vi "TestCloneAPI.vi"() -> ()   [LabVIEW 2014, in "DigitizerModule.lvlib"]
uses:
  DigitizerModule.lvlib
  DigitizerPlugins/DigitizerBaseClass/Typedefs/WfrmAttributes.ctl
  TestInfo.ctl
  <userlib>/NIST/ModuleAdminLib/CloneRegistration/CloneRegistration.lvclass
  <userlib>/NIST/ModuleAdminLib/ModuleAdmin/ModuleAdmin.lvclass/ModuleAdmin.ctl
  <userlib>/NIST/ModuleAdminLib/ModuleAdmin/ModuleAdmin.lvclass
  PublicAPI/Arguments/Broadcasts/clDidInit.ctl
  PublicAPI/Arguments/Requests/clStopArgument.ctl
  <userlib>/NIST/ModuleAdminLib/ModuleAdmin/Accessors/Read CloneRegRef.vi
  <userlib>/NIST/ModuleAdminLib/ModuleAdmin/Accessors/Write CloneRegRef.vi
  DigitizerPlugins/DigitizerBaseClass/DigitizerBase.lvclass
panel:
  out "Attributes":T1[][](array[typedef])
  out "Timing":cluster{"Time Stamp":timestamp, "dt":dbl}[][](array[cluster])
  in  "btnAbort":bool
  in  "btnClear":bool
  in  "btnCfgTrig":bool
  in  "btnCfgAquis":bool
  in  "btnCfgChan":bool
  out "Waveform Chart":waveform(dbl)[](graph)
  in  "btnInitialize":bool
  in  "btnReadWfrm":bool
  in  "btnFetch":bool
  in  "btnPref":bool
  in  "Show Panel":bool=TRUE
  in  "Plugin Type":u16(ring) items=["IVI Digitizer", "Analyse Waveforms", "Debug", "Ni DaqMx Digitizer", "PMU Cal", "(obsolete)", "Simulation"]
  in  "btnLoadPlugin":bool
  out "Path":path
  in  "btnRequestINIPath":bool
  in  "btnRemove":bool
  out "Status Log":string
  out "Active Modules (Array)":string[](array[string])
  in  "btnAdd":bool
  in  "btnStop":bool
  in  "Select Module":i32(ring)=-1 caption="Select Module to send Request" items=["All"=-1, "4140002"=4140002]
  # "Hidden"
  # "Visible"
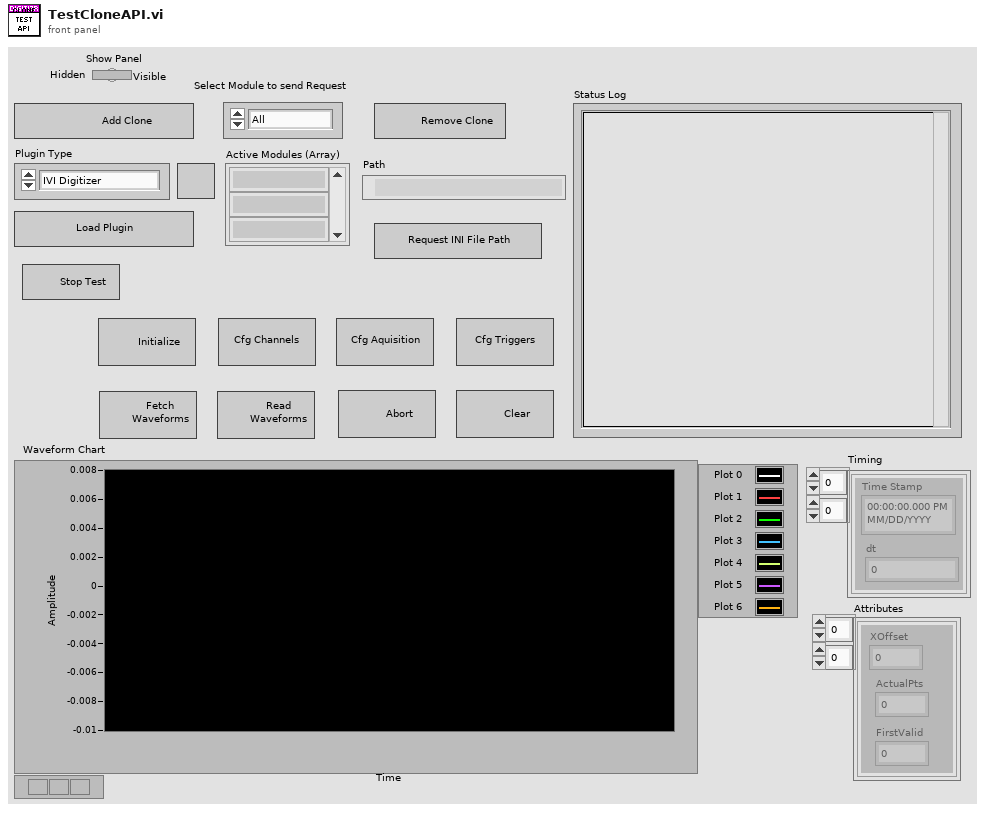
[diagram p1: front panel]
types:
  T1 = typedef "DigitizerPlugins.lvlib/DigitizerBase.lvclass/WfrmAttributes.ctl" = cluster{"XOffset":dbl, "ActualPts":i64, "FirstValid":i64}
  T2 = typedef "DigitizerModule.lvlib/TestInfo.ctl" = cluster{"PluginIniFilePaths":path[]}
  T3 = typedef "DigitizerModule.lvlib/clBroadcastEvents.ctl" = cluster{"DidInit":refnum<user-event>, "StatusUpdate":refnum<user-event>, "ErrorReport":refnum<user-event>, "DidStop":refnum<user-event>, "PathToINI":refnum<user-event>, "Channels":refnum<user-event>, "Acq":refnum<user-event>, "Trigger":refnum<user-event>, "Waveforms":refnum<user-event>}
  T4 = typedef "DigitizerModule.lvlib/clDidInit.ctl" = cluster{"Init?":bool, "ModuleAdmin":refnum<class "ModuleAdmin.lvclass">}
  T5 = typedef "DigitizerModule.lvlib/clStopArgument.ctl" = cluster{"Exit via Stop Module Req?":bool, "Wait for Module to stop?":bool, "ModuleAdmin":refnum<class "ModuleAdmin.lvclass">}
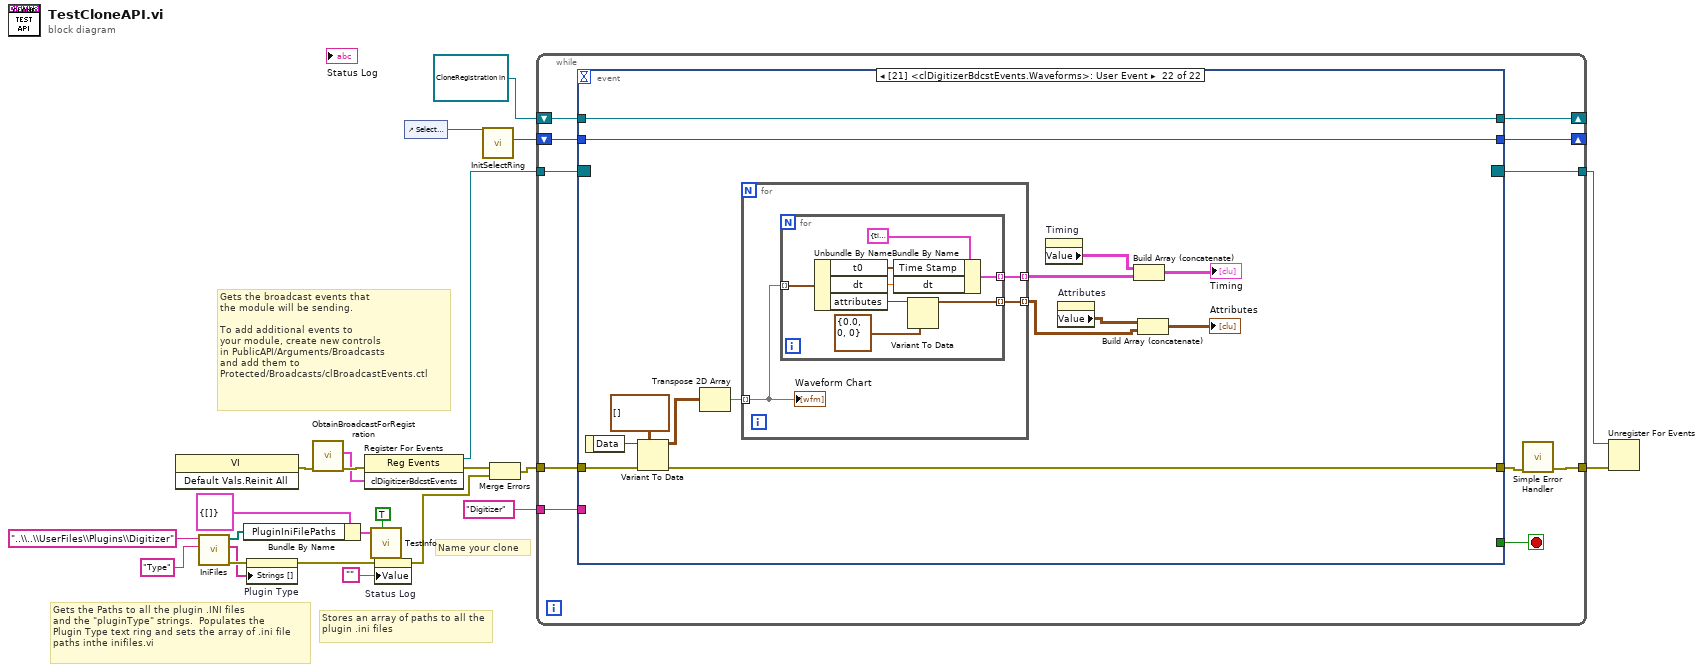
[diagram p0: block diagram]
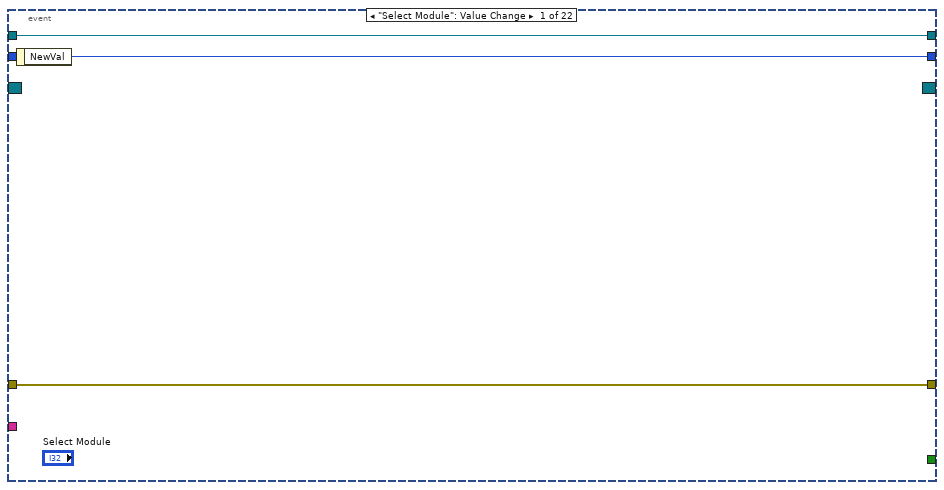
[diagram p2: hidden frame]
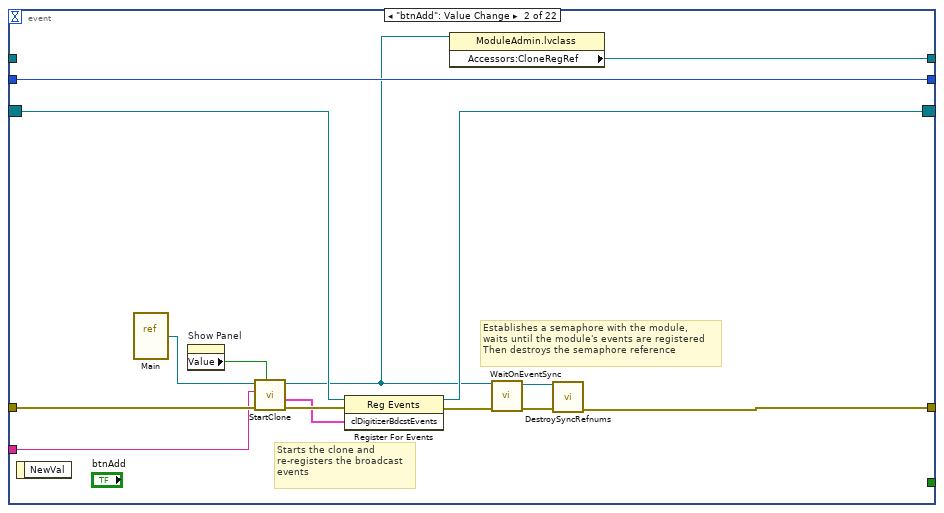
[diagram p3: hidden frame]
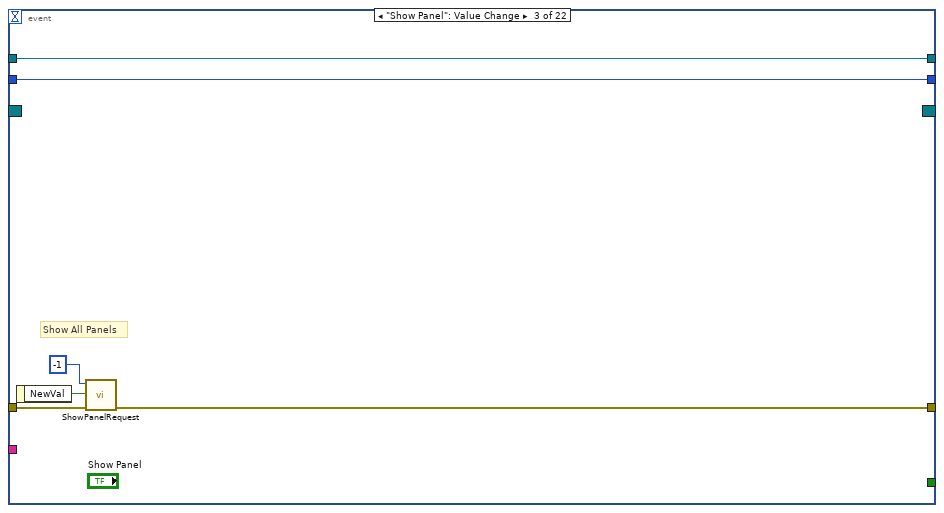
[diagram p4: hidden frame]
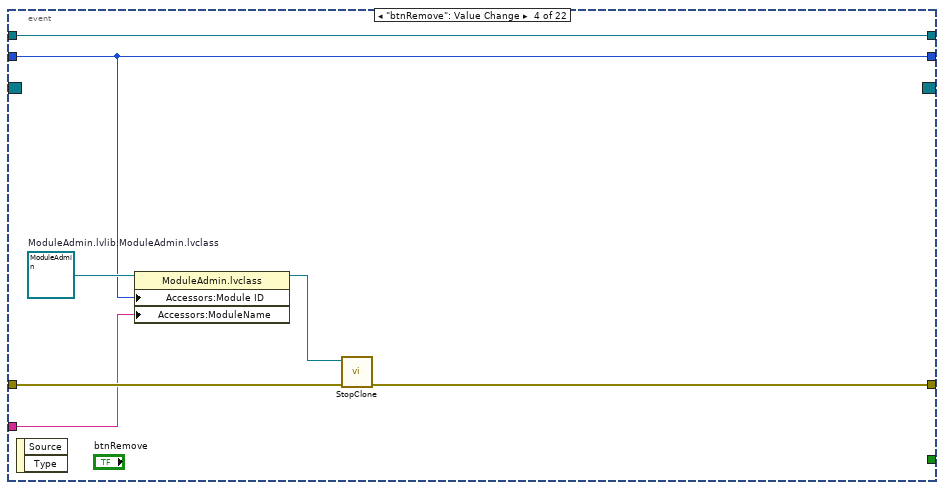
[diagram p5: hidden frame]
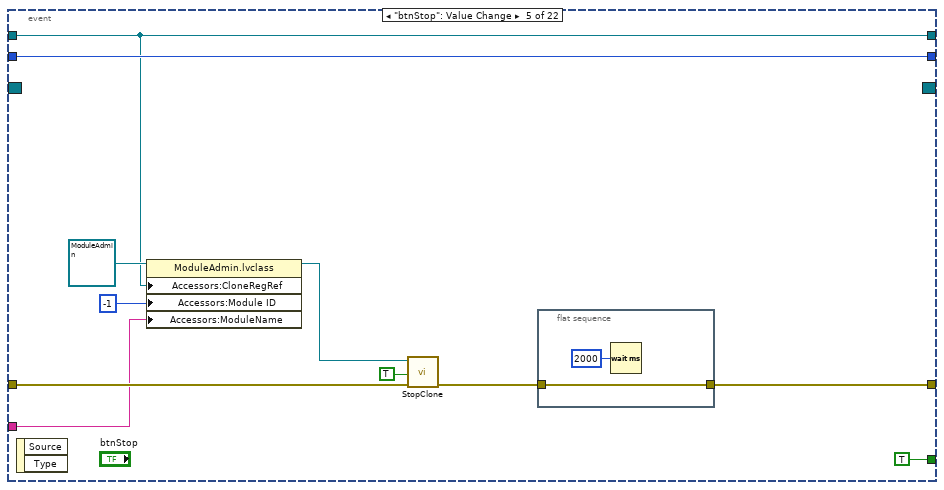
[diagram p6: hidden frame]
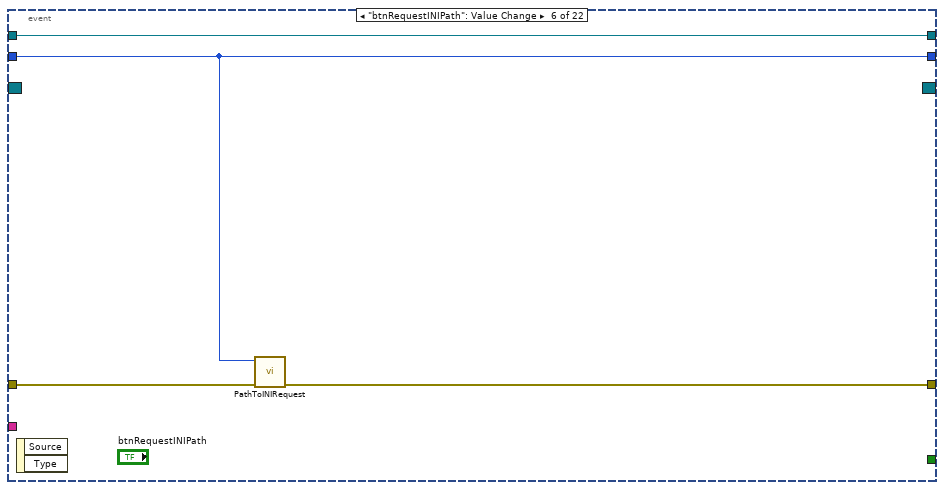
[diagram p7: hidden frame]
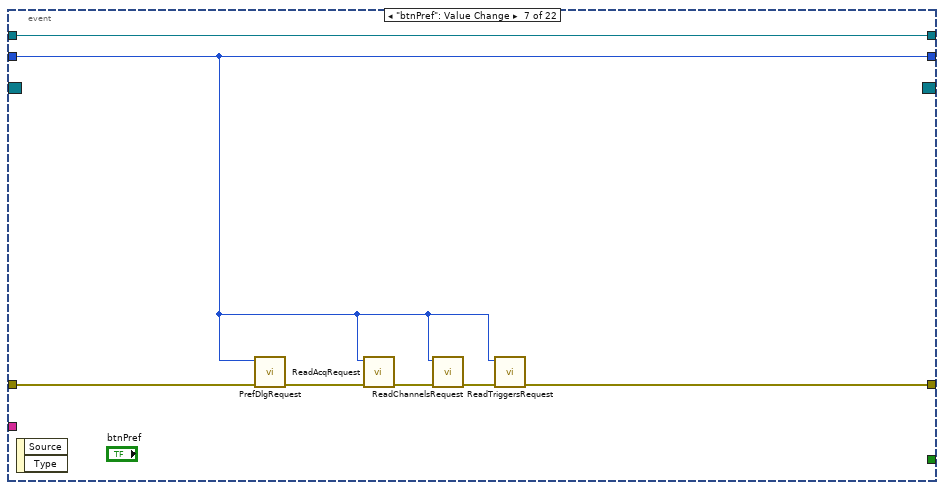
[diagram p8: hidden frame]
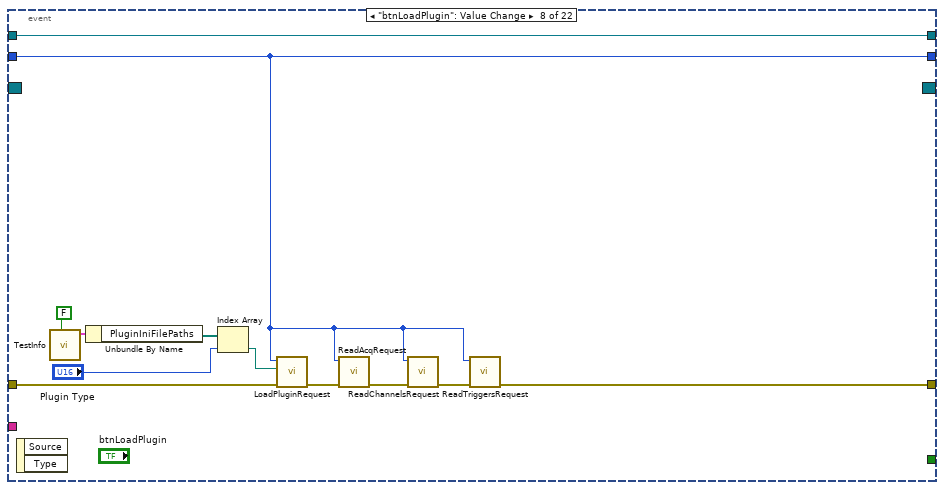
[diagram p9: hidden frame]
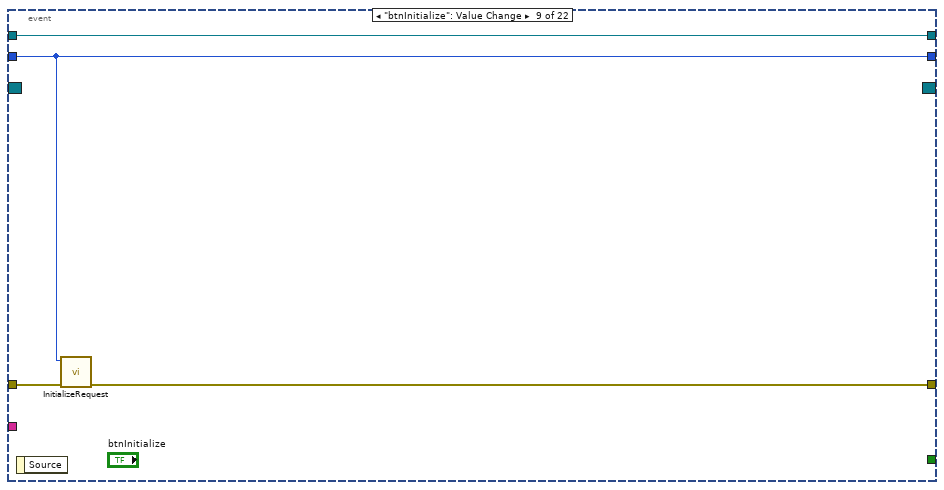
[diagram p10: hidden frame]
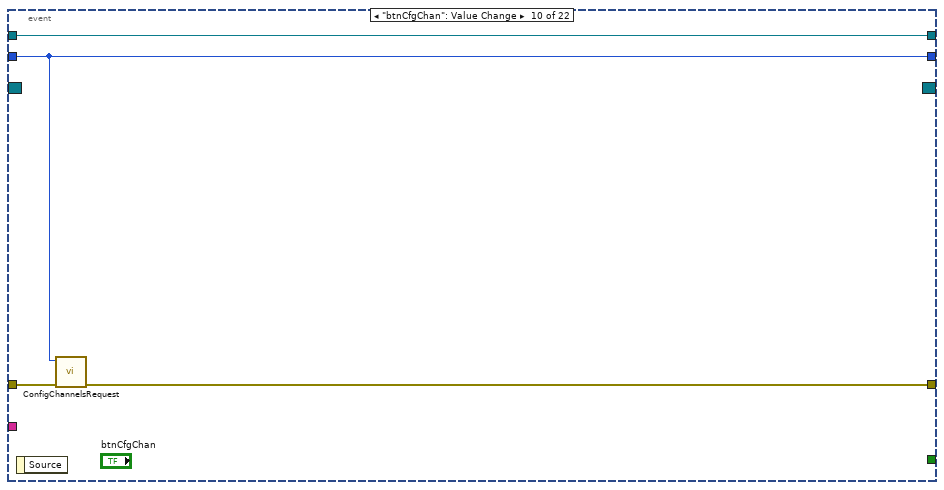
[diagram p11: hidden frame]
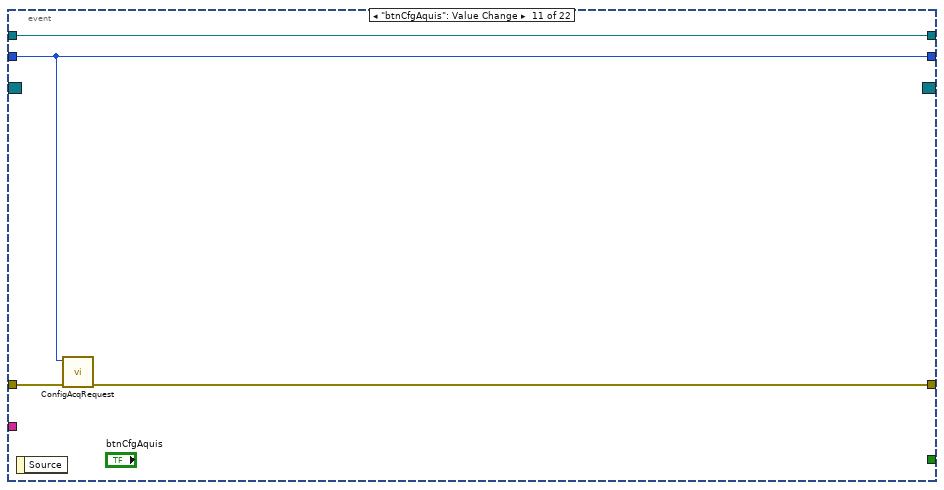
[diagram p12: hidden frame]
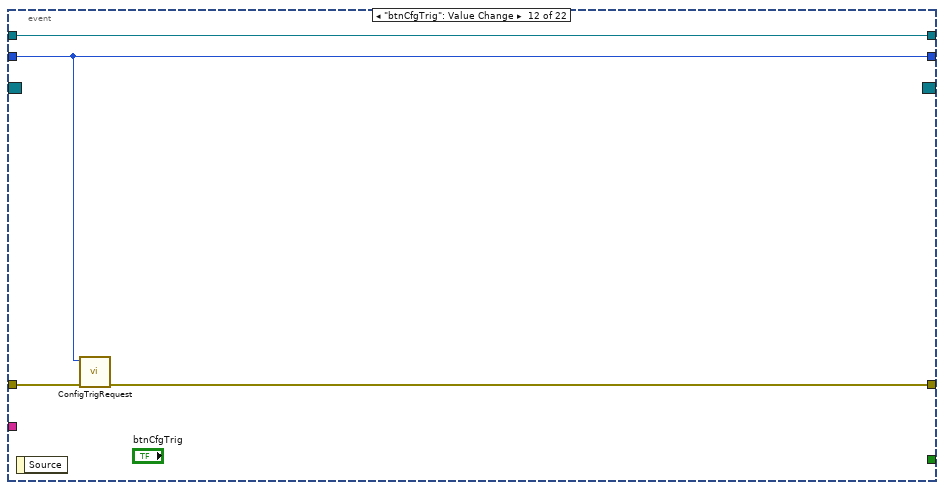
[diagram p13: hidden frame]
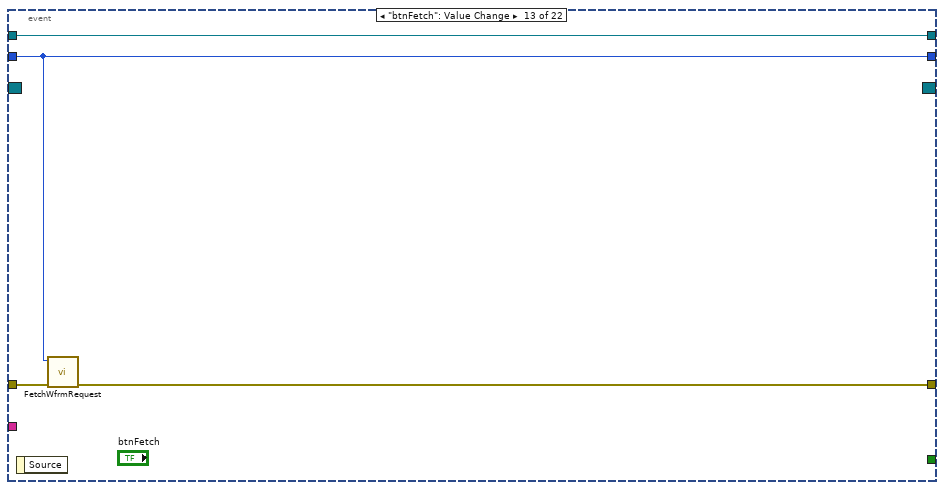
[diagram p14: hidden frame]
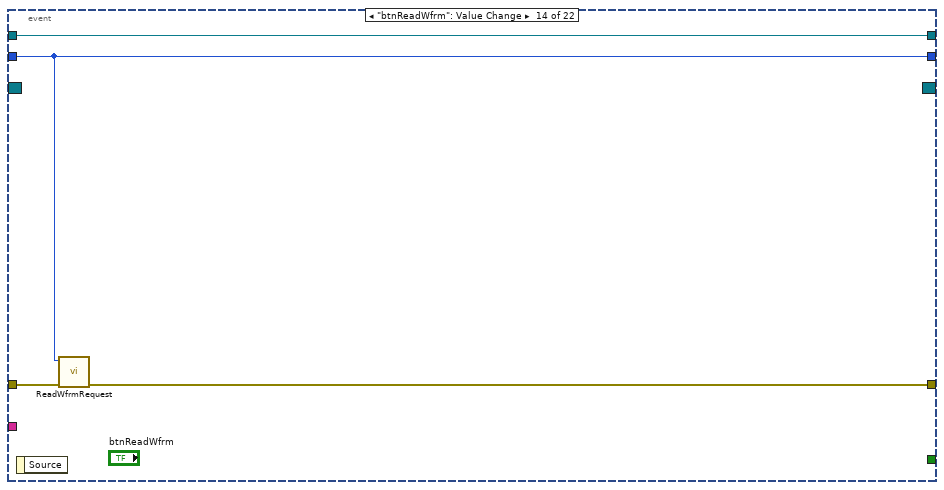
[diagram p15: hidden frame]
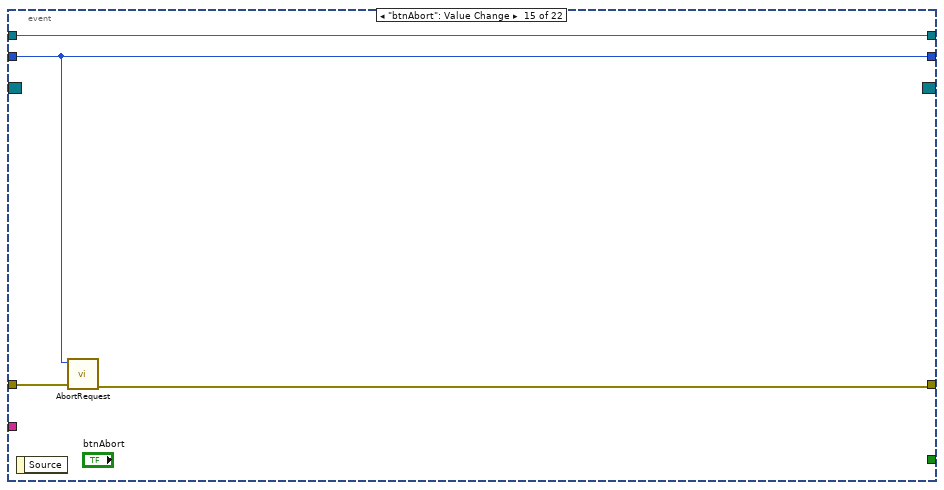
[diagram p16: hidden frame]
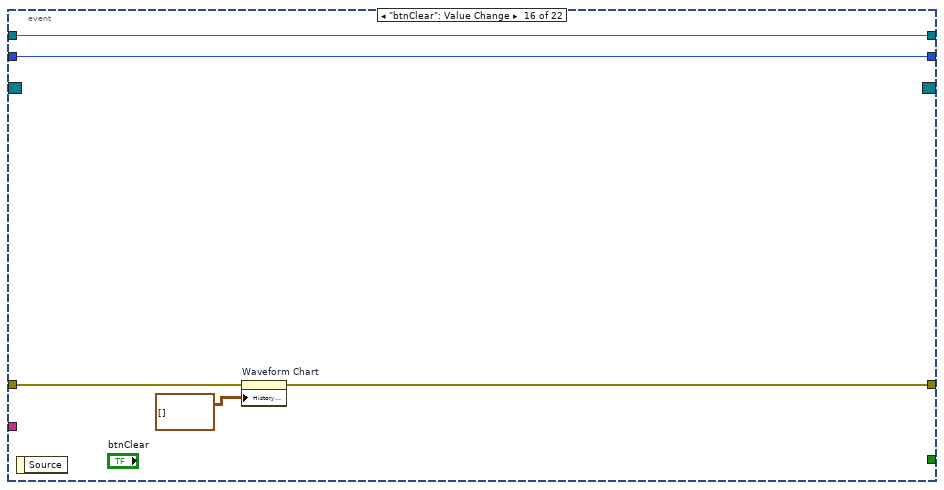
[diagram p17: hidden frame]
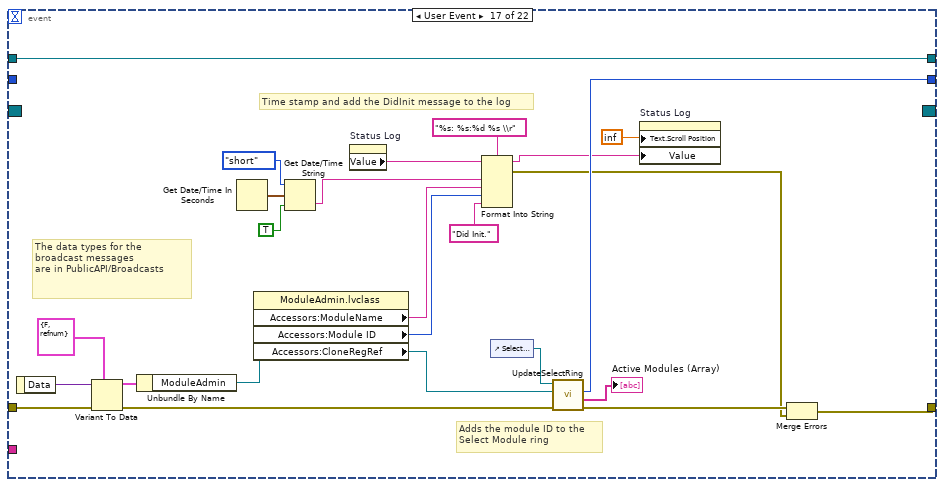
[diagram p18: hidden frame]
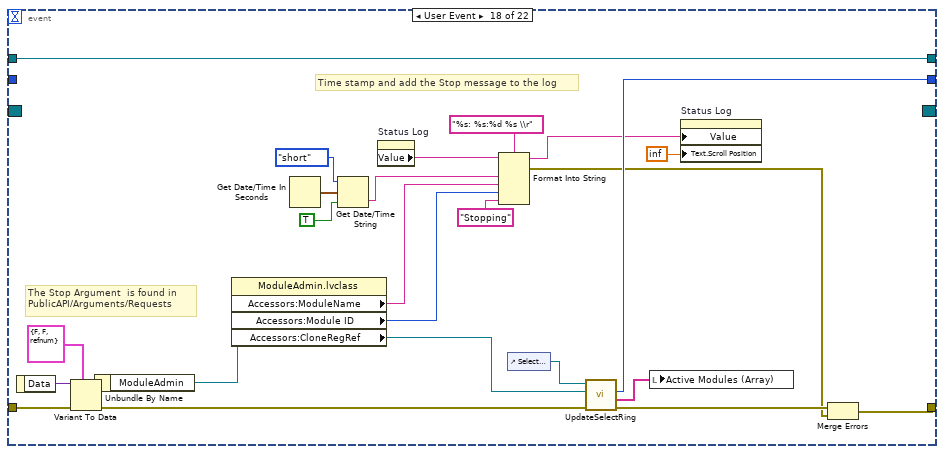
[diagram p19: hidden frame]
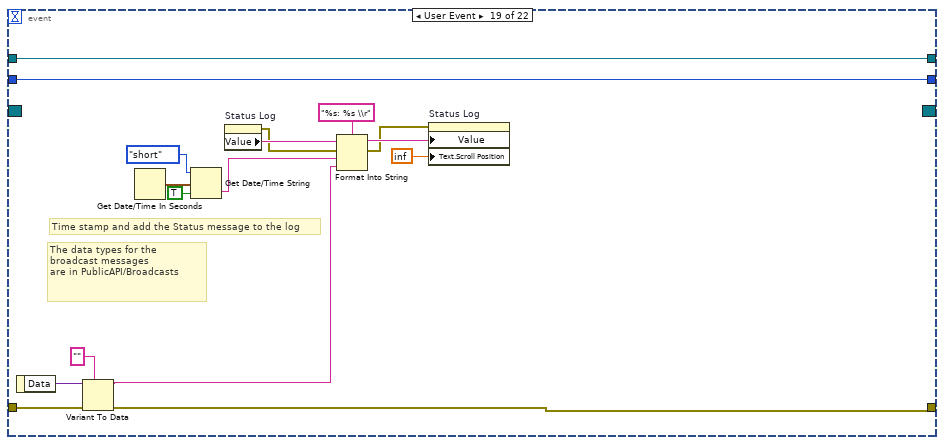
[diagram p20: hidden frame]
diagram:
  # "Stores an array of paths to all the plugin .ini files"
  # "Gets the Paths to all the plugin .INI files\nand the \"pluginType\" strings.  Populates the \nPlugin Type text ring and sets the array of .ini file\npaths inthe inifiles.vi"
  # "Name your clone"
  # "Gets the broadcast events that\nthe module will be sending.\n\nTo add additional events to\nyour module, create new controls\nin PublicAPI/Arguments/Broadcasts\nand add them to\nProtected/Broadcasts/clBroadcastEvents.ctl"
  n1 = invoke class="VI" method="Default Vals.Reinit All"() -> (error out=w21:errorcluster)  [unwired: 3 in, 2 out]
  n2 = call "IniFiles.vi"("iniKey"="Type", "name or relative path"="..\\..\\UserFiles\\Plugins\\Digitizer") -> ("error out"=w15:errorcluster, "Types"=w14:string[], "IniFilePaths"=w13:path[])  [unwired: 7 in]
  n3 = Bundle By Name(cluster=T2 {"PluginIniFilePaths"=[]} ("TestInfo"), "PluginIniFilePaths"=w13) -> (w12:T2)
  n4 = property on="Plugin Type" class="Ring (strict)"(error in=w15, "Strings []"=w14) -> (error out=w3:errorcluster)  [unwired: 1 in, 1 out]
  n5 = call "ObtainBroadcastForRegistration.vi"("error in (no error)"=w21) -> ("error out"=w20:errorcluster, "clDigitizerBdcstEvents"=w19:T3)  [unwired: 9 in]
  n6 = register-events(error in=w20, w19) -> (reference out=w17:refnum<event-registration>, error out=w18:errorcluster)  [unwired: 1 in]
  n7 = call "TestInfo.vi"("Set (f)"=TRUE, "TestInfo 2"=w12) -> ()  [unwired: 9 in, 1 out]
  n8 = property on="Status Log" class="Str"(error in=w3, "Value"="") -> (error out=w2:errorcluster)  [unwired: 1 in, 1 out]
  n9 = control-ref of="Select Module"() -> (w23:refnum<vi>)
  n10 = call "InitSelectRing.vi"("Ring Refnum"=w23) -> ("Module Ring Value"=w22:i32)  [unwired: 9 in, 1 out]
  n11 = Merge Errors(w18, w2) -> (w10:errorcluster)
  n12 = while {
    shift-right: [w33] -> _
    shift-left: w22 -> [w34]
    tunnel: w10 -> [w31]
    tunnel: w17 -> [w28]
    tunnel: [w29] -> w6
    tunnel: "Digitizer" ("ModuleName") -> [w27]
    tunnel: [w26] -> w5
    shift-right: [w25] -> _
    shift-left: refnum<data-value> refnum ("Accessors:CloneRegRef") -> [w24]
    stop <- w32 stop-if-true
    n13 = event shown="[21] <clDigitizerBdcstEvents.Waveforms>: User Event" {
      selector: w28 -> [_ w44 _ _ _ _ _ _ _ _ _ _ _ _ _ _ _ _ _ _ _ _]
      dyn-events: [_ w43 _ _ _ _ _ _ _ _ _ _ _ _ _ _ _ _ _ _ _ _] -> w26
      timeout: _ -> [_ _ _ _ _ _ _ _ _ _ _ _ _ _ _ _ _ _ _ _ _ _]
      tunnel: w34 -> [_ w52 w54 w62 w76 w82 w83 w90 w102 w108 w112 w114 w118 w122 w128 w133 _ _ w201 w204 w217 w226]
      tunnel: [w37 w52 w54 w62 w76 w82 w83 w90 w102 w108 w112 w114 w118 w122 w128 w133 w154 w173 w201 w204 w217 w226] -> w33
      tunnel: [_ _ _ _ TRUE _ _ _ _ _ _ _ _ _ _ _ _ _ _ _ _ _] -> w32
      tunnel: w31 -> [w36 w51 w57 w65 w74 w81 w89 w101 w105 w109 w113 w116 w121 w125 w129 w132 w159 w180 w199 w209 w213 w230]
      tunnel: [w36 w45 w55 w64 w66 w80 w84 w91 w104 w106 w110 w115 w120 w124 w126 w131 w145 w170 w185 w208 w212 w228] -> w30
      tunnel: w27 -> [_ w41 _ w61 w71 _ _ _ _ _ _ _ _ _ _ _ _ _ _ _ _ _]
      tunnel: [w35 w38 w53 w59 w68 w79 w88 w95 w103 w107 w111 w117 w119 w123 w127 w134 w138 w163 w191 w202 w211 w227] -> w25
      tunnel: w24 -> [w35 _ w53 w59 w68 w79 w88 w95 w103 w107 w111 w117 w119 w123 w127 w134 w138 w163 w191 w202 w211 w227]
      event "Select Module": Value Change {
        n14 = event-data() -> ("NewVal"=w37:i32)  [unwired: 1 in]
      }
      event "btnAdd": Value Change {
        # "Establishes a semaphore with the module,\nwaits until the module's events are registered\nThen destroys the semaphore reference"
        # "Starts the clone and\nre-registers the broadcast \nevents"
        n15 = event-data() -> ()  [unwired: 1 in, 1 out]
        n16 = vi-ref "Main.vi"() -> (w42:refnum<vi>)
        n17 = property on="Show Panel" class="Bool (strict)"() -> ("Value"=w40:bool)  [unwired: 2 in, 2 out]
        n18 = call "StartClone.vi"("ShowPanel? (f)"=w40, "error in (no error)"=w51, "ModuleName"=w41, "VI Refnum"=w42) -> ("error out"=w50:errorcluster, "clBroadcastEvents"=w46:T3, "ModuleAdmin"=w39:refnum<class "ModuleAdmin.lvclass">)  [unwired: 5 in]
        n19 = register-events(reference=w44, error in=w50, w46) -> (reference out=w43:refnum<event-registration>, error out=w49:errorcluster)
        n20 = property class="ModuleAdmin.lvclass"(reference=w39) -> ("Accessors:CloneRegRef"=w38:refnum<data-value>)  [unwired: 1 in, 2 out]
        n21 = call <userlib>:"WaitOnEventSync.vi"("error in (no error)"=w49, "ModuleAdmin"=w39) -> ("error out"=w48:errorcluster, "ModuleAdmin"=w47:refnum<class "ModuleAdmin.lvclass">)  [unwired: 8 in]
        n22 = call <userlib>:"DestroySyncRefnums.vi"("error in (no error)"=w48, "ModuleAdmin"=w47) -> ("error out"=w45:errorcluster)  [unwired: 9 in]
      }
      event "Show Panel": Value Change {
        # "Show All Panels"
        n23 = event-data() -> ("NewVal"=w58:bool)  [unwired: 1 in]
        n24 = call "ShowPanelRequest.vi"("error in (no error)"=w57, "ShowPanel?"=w58, "ModuleID"=-1) -> ("error out"=w55:errorcluster)  [unwired: 8 in]
      }
      event "btnRemove": Value Change {
        w63 = refnum<class "ModuleAdmin.lvclass"> refnum  # ModuleAdmin.lvlib:ModuleAdmin.lvclass
        n25 = event-data() -> ()  [unwired: 1 in, 2 out]
        n26 = property class="ModuleAdmin.lvclass"(reference=w63, "Accessors:Module ID"=w62, "Accessors:ModuleName"=w61) -> (reference out=w60:refnum<class "ModuleAdmin.lvclass">)  [unwired: 1 in, 1 out]
        n27 = call "StopClone.vi"("error in (no error)"=w65, "ModuleAdmin"=w60) -> ("error out"=w64:errorcluster)  [unwired: 9 in]
      }
      event "btnStop": Value Change {
        n28 = event-data() -> ()  [unwired: 1 in, 2 out]
        n29 = property class="ModuleAdmin.lvclass"(reference=refnum<class "ModuleAdmin.lvclass"> refnum ("ModuleAdmin.lvlib:ModuleAdmin.lvclass"), "Accessors:CloneRegRef"=w68, "Accessors:Module ID"=-1 ("Module ID"), "Accessors:ModuleName"=w71) -> (reference out=w70:refnum<class "ModuleAdmin.lvclass">)  [unwired: 1 in, 1 out]
        n30 = call "StopClone.vi"("error in (no error)"=w74, "Wait for Module to stop?"=TRUE, "ModuleAdmin"=w70) -> ("error out"=w67:errorcluster)  [unwired: 8 in]
        n31 = flat-sequence {
          tunnel: w67 -> [w77]
          tunnel: [w77] -> w66
          frame #0 {
            n32 = Wait (ms)(milliseconds to wait=u32 2000) -> ()  [unwired: 1 out]
          }
        }
      }
      event "btnRequestINIPath": Value Change {
        n33 = event-data() -> ()  [unwired: 1 in, 2 out]
        n34 = call "PathToINIRequest.vi"("error in (no error)"=w81, "ModuleID"=w82) -> ("error out"=w80:errorcluster)  [unwired: 9 in]
      }
      event "btnPref": Value Change {
        n35 = event-data() -> ()  [unwired: 1 in, 2 out]
        n36 = call "PrefDlgRequest.vi"("error in (no error)"=w89, "ModuleID"=w83) -> ("error out"=w87:errorcluster)  [unwired: 9 in]
        n37 = call "ReadAcqRequest.vi"("error in (no error)"=w87, "ModuleID"=w83) -> ("error out"=w86:errorcluster)  [unwired: 9 in]
        n38 = call "ReadChannelsRequest.vi"("error in (no error)"=w86, "ModuleID"=w83) -> ("error out"=w85:errorcluster)  [unwired: 9 in]
        n39 = call "ReadTriggersRequest.vi"("error in (no error)"=w85, "ModuleID"=w83) -> ("error out"=w84:errorcluster)  [unwired: 9 in]
      }
      event "btnLoadPlugin": Value Change {
        n40 = event-data() -> ()  [unwired: 1 in, 2 out]
        n41 = call "TestInfo.vi"("Set (f)"=FALSE) -> ("TestInfo"=w99:T2)  [unwired: 10 in]
        n42 = Unbundle By Name(w99) -> ("PluginIniFilePaths"=w98:path[])
        n43 = Index Array(array=w98, index="Plugin Type") -> (element=w96:path)
        n44 = call "LoadPluginRequest.vi"("error in (no error)"=w101, "PathToPluginINI"=w96, "ModuleID"=w90) -> ("error out"=w94:errorcluster)  [unwired: 8 in]
        n45 = call "ReadAcqRequest.vi"("error in (no error)"=w94, "ModuleID"=w90) -> ("error out"=w93:errorcluster)  [unwired: 9 in]
        n46 = call "ReadChannelsRequest.vi"("error in (no error)"=w93, "ModuleID"=w90) -> ("error out"=w92:errorcluster)  [unwired: 9 in]
        n47 = call "ReadTriggersRequest.vi"("error in (no error)"=w92, "ModuleID"=w90) -> ("error out"=w91:errorcluster)  [unwired: 9 in]
      }
      event "btnInitialize": Value Change {
        n48 = event-data() -> ()  [unwired: 1 in, 1 out]
        n49 = call "InitializeRequest.vi"("error in (no error)"=w105, "ModuleID"=w102) -> ("error out"=w104:errorcluster)  [unwired: 9 in]
      }
      event "btnCfgChan": Value Change {
        n50 = event-data() -> ()  [unwired: 1 in, 1 out]
        n51 = call "ConfigChannelsRequest.vi"("error in (no error)"=w109, "ModuleID"=w108) -> ("error out"=w106:errorcluster)  [unwired: 9 in]
      }
      event "btnCfgAquis": Value Change {
        n52 = event-data() -> ()  [unwired: 1 in, 1 out]
        n53 = call "ConfigAcqRequest.vi"("error in (no error)"=w113, "ModuleID"=w112) -> ("error out"=w110:errorcluster)  [unwired: 9 in]
      }
      event "btnCfgTrig": Value Change {
        n54 = event-data() -> ()  [unwired: 1 in, 1 out]
        n55 = call "ConfigTrigRequest.vi"("error in (no error)"=w116, "ModuleID"=w114) -> ("error out"=w115:errorcluster)  [unwired: 9 in]
      }
      event "btnFetch": Value Change {
        n56 = event-data() -> ()  [unwired: 1 in, 1 out]
        n57 = call "FetchWfrmRequest.vi"("error in (no error)"=w121, "ModuleID"=w118) -> ("error out"=w120:errorcluster)  [unwired: 9 in]
      }
      event "btnReadWfrm": Value Change {
        n58 = event-data() -> ()  [unwired: 1 in, 1 out]
        n59 = call "ReadWfrmRequest.vi"("error in (no error)"=w125, "ModuleID"=w122) -> ("error out"=w124:errorcluster)  [unwired: 9 in]
      }
      event "btnAbort": Value Change {
        n60 = event-data() -> ()  [unwired: 1 in, 1 out]
        n61 = call "AbortRequest.vi"("error in (no error)"=w129, "ModuleID"=w128) -> ("error out"=w126:errorcluster)  [unwired: 9 in]
      }
      event "btnClear": Value Change {
        n62 = event-data() -> ()  [unwired: 1 in, 1 out]
        n63 = property on="Waveform Chart" class="WFChart (strict)"(error in=w132, "History Data"=waveform(dbl)[][] []) -> (error out=w131:errorcluster)  [unwired: 1 in, 1 out]
      }
      event User Event {
        # "Adds the module ID to the \nSelect Module ring"
        # "Time stamp and add the DidInit message to the log"
        # "The data types for the broadcast messages\nare in PublicAPI/Broadcasts"
        n64 = event-data() -> ("Data"=w158:variant)  [unwired: 1 in]
        n65 = Variant To Data(error in=w159, type=T4 {"Init?"=FALSE, "ModuleAdmin"=refnum} ("clDidInit"), Variant=w158) -> (data=w151:T4, error out=w156:errorcluster)
        n66 = Unbundle By Name(w151) -> ("ModuleAdmin"=w143:refnum<class "ModuleAdmin.lvclass">)
        n67 = Get Date/Time In Seconds() -> (seconds since 1Jan1904=w149:timestamp)
        n68 = property class="ModuleAdmin.lvclass"(reference=w143) -> ("Accessors:ModuleName"=w141:string, "Accessors:Module ID"=w140:i32, "Accessors:CloneRegRef"=w139:refnum<data-value>)  [unwired: 1 in, 2 out]
        n69 = Get Date/Time String(date format (0)=enum16{"short", "long", "abbreviated"}."short", seconds (now)=w149, want seconds? (F)=TRUE) -> (time string=w152:string)  [unwired: 1 out]
        n70 = property on="Status Log" class="Str"() -> ("Value"=w137:string)  [unwired: 2 in, 2 out]
        n71 = Format Into String(format string="%s: %s:%d %s \\r", initial string=w137, w152, w141, w140, "Did Init.") -> (resulting string=w136:string, error out=w146:errorcluster)  [unwired: 1 in]
        n72 = control-ref of="Select Module"() -> (w155:refnum<vi>)
        n73 = call "UpdateSelectRing.vi"("error in (no error)"=w156, "CloneRegRef"=w139, "Ring Refnum"=w155) -> ("error out"=w147:errorcluster, "ActiveModules"=→"Active Modules (Array)":string[], "Module Ring Value"=w154:i32)  [unwired: 6 in]
        n74 = property on="Status Log" class="Str"("Text.Scroll Position"=inf, "Value"=w136) -> ()  [unwired: 2 in, 2 out]
        n75 = Merge Errors(w147, w146) -> (w145:errorcluster)
      }
      event User Event {
        # "Time stamp and add the Stop message to the log"
        # "The Stop Argument  is found in\nPublicAPI/Arguments/Requests"
        n76 = event-data() -> ("Data"=w179:variant)  [unwired: 1 in]
        n77 = Variant To Data(error in=w180, type=T5 {"Exit via Stop Module Req?"=FALSE, "Wait for Module to stop?"=FALSE, "ModuleAdmin"=refnum} ("Stop Argument"), Variant=w179) -> (data=w177:T5, error out=w176:errorcluster)
        n78 = Unbundle By Name(w177) -> ("ModuleAdmin"=w168:refnum<class "ModuleAdmin.lvclass">)
        n79 = property class="ModuleAdmin.lvclass"(reference=w168) -> ("Accessors:ModuleName"=w166:string, "Accessors:Module ID"=w165:i32, "Accessors:CloneRegRef"=w164:refnum<data-value>)  [unwired: 1 in, 2 out]
        n80 = Get Date/Time In Seconds() -> (seconds since 1Jan1904=w182:timestamp)
        n81 = Get Date/Time String(date format (0)=enum16{"short", "long", "abbreviated"}."short", seconds (now)=w182, want seconds? (F)=TRUE) -> (time string=w184:string)  [unwired: 1 out]
        n82 = property on="Status Log" class="Str"() -> ("Value"=w162:string)  [unwired: 2 in, 2 out]
        n83 = Format Into String(format string="%s: %s:%d %s \\r", initial string=w162, w184, w166, w165, "Stopping") -> (resulting string=w161:string, error out=w171:errorcluster)  [unwired: 1 in]
        n84 = control-ref of="Select Module"() -> (w175:refnum<vi>)
        n85 = call "UpdateSelectRing.vi"("error in (no error)"=w176, "CloneRegRef"=w164, "Ring Refnum"=w175) -> ("error out"=w172:errorcluster, "ActiveModules"=w174:string[], "Module Ring Value"=w173:i32)  [unwired: 6 in]
        n86 = local write "Active Modules (Array)"(w174) -> ()
        n87 = property on="Status Log" class="Str"("Value"=w161, "Text.Scroll Position"=inf) -> ()  [unwired: 2 in, 2 out]
        n88 = Merge Errors(w172, w171) -> (w170:errorcluster)
      }
      event User Event {
        # "Time stamp and add the Status message to the log"
        # "The data types for the broadcast messages\nare in PublicAPI/Broadcasts"
        n89 = event-data() -> ("Data"=w198:variant)  [unwired: 1 in]
        n90 = Variant To Data(error in=w199, type="" ("clStatUpdate"), Variant=w198) -> (data=w192:string, error out=w185:errorcluster)
        n91 = Get Date/Time In Seconds() -> (seconds since 1Jan1904=w196:timestamp)
        n92 = Get Date/Time String(date format (0)=enum16{"short", "long", "abbreviated"}."short", seconds (now)=w196, want seconds? (F)=TRUE) -> (time string=w193:string)  [unwired: 1 out]
        n93 = property on="Status Log" class="Str"() -> (error out=w188:errorcluster, "Value"=w190:string)  [unwired: 2 in, 1 out]
        n94 = Format Into String(format string="%s: %s \\r", initial string=w190, error in=w188, w193, w192) -> (resulting string=w189:string, error out=w187:errorcluster)
        n95 = property on="Status Log" class="Str"(error in=w187, "Value"=w189, "Text.Scroll Position"=inf) -> ()  [unwired: 1 in, 2 out]
      }
      event User Event {
        # "#CodeNeeded\nThis is a very crude error handler\nA better error handler will be needed"
        # "The data types for the broadcast messages\nare in PublicAPI/Broadcasts"
        n96 = event-data() -> ("ModuleID"=w206:i32, "Data"=w210:variant)  [unwired: 1 in]
        n97 = Variant To Data(error in=w209, type=errorcluster {"status"=FALSE, "code"=0, "source"=""} ("Cluster"), Variant=w210) -> (data=w203:errorcluster, error out=w208:errorcluster)
        n98 = Number To Decimal String(number=w206) -> (decimal integer string=w205:string)  [unwired: 1 in]
        n99 = call <vilib>:"General Error Handler.vi"("[error source] (\" \")"=w205, "error in (no error)"=w203) -> ()  [unwired: 9 in, 5 out]
      }
      event User Event {
        n100 = event-data() -> ("Data"=w215:variant)  [unwired: 1 in, 1 out]
        n101 = Variant To Data(error in=w213, type=path "" ("Path"), Variant=w215) -> (data=→"Path":path, error out=w212:errorcluster)
      }
      event User Event {
        n102 = event-data() -> ("Data"=w231:variant)  [unwired: 1 in]
        n103 = Variant To Data(error in=w230, type=waveform(dbl)[][] [], Variant=w231) -> (data=w225:waveform(dbl)[][], error out=w228:errorcluster)
        n104 = Transpose 2D Array(2D array=w225) -> (transposed array=w224:waveform(dbl)[][])
        n105 = for {
          tunnel: w224 -> [w234] mode=indexing
          tunnel: [w233] -> w219 mode=indexing
          tunnel: [w232] -> w222 mode=indexing
          n106 = for {
            tunnel: w234 -> [w242] mode=indexing
            tunnel: [w236] -> w232 mode=indexing
            tunnel: [w235] -> w233 mode=indexing
            n107 = Unbundle By Name(w242) -> ("t0"=w240:timestamp, "dt"=w239:dbl, "attributes"=w238:variant)
            n108 = Bundle By Name(cluster=cluster{"Time Stamp":timestamp, "dt":dbl} {"Time Stamp"=timestamp(0 s since 1904-01-01), "dt"=0.0} ("Cluster"), "Time Stamp"=w240, "dt"=w239) -> (w236:cluster{"Time Stamp":timestamp, "dt":dbl})
            n109 = Variant To Data(type=T1 {"XOffset"=0.0, "ActualPts"=0, "FirstValid"=0} ("Attributes"), Variant=w238) -> (data=w235:T1)  [unwired: 1 in, 1 out]
          }
          "Waveform Chart" <- w234
        }
        n110 = property on="Timing" class="Arr (strict)"() -> ("Value"=w223:cluster{"Time Stamp":timestamp, "dt":dbl}[][])  [unwired: 2 in, 2 out]
        n111 = property on="Attributes" class="Arr (strict)"() -> ("Value"=w220:T1[][])  [unwired: 2 in, 2 out]
        n112 = Build Array (concatenate)(w223, w222) -> (→"Timing":cluster{"Time Stamp":timestamp, "dt":dbl}[][])
        n113 = Build Array (concatenate)(w220, w219) -> (→"Attributes":T1[][])
      }
    }
    n114 = call <vilib>:"Simple Error Handler.vi"("error in (no error)"=w30) -> ("error out"=w29:errorcluster)  [unwired: 4 in, 4 out]
  }
  n115 = Unregister For Events(event registration refnum=w5, error in=w6) -> ()  [unwired: 1 out]
